vi "light_control.vi"() -> ()   [LabVIEW 2017]
uses:
  <vilib>/LabVIEW Interface for Arduino/Type Defs/Arduino Resource.ctl
  <vilib>/LabVIEW Interface for Arduino/Type Defs/Board Type.ctl
  <vilib>/LabVIEW Interface for Arduino/LabVIEW Interface for Arduino.lvlib
panel:
  in  "紫光":bool
  in  "PWM9":u8=70
  in  "PWM8":u8=70
  in  "PWM7":u8=70
  in  "PWM6":u8=70
  in  "PWM4":u8=70
  in  "PWM5":u8=70
  in  "PWM1":u8=70
  in  "PWM3":u8=70
  in  "PWM2":u8=70
  out "PWM Pins 3":u8[](array[numeric])
  out "PWM Pins 2":u8[](array[numeric])
  out "PWM Pins":u8[](array[numeric])
  out "机电控制报错1":errorcluster caption="机电控制报错"
  out "机电控制资源1":T1={"VISA resource"="", "Board Type"=enum."Uno", "Connection Type"=enum."USB / Serial", "Bytes Per Packet (15)"=15} caption="机电控制资源"
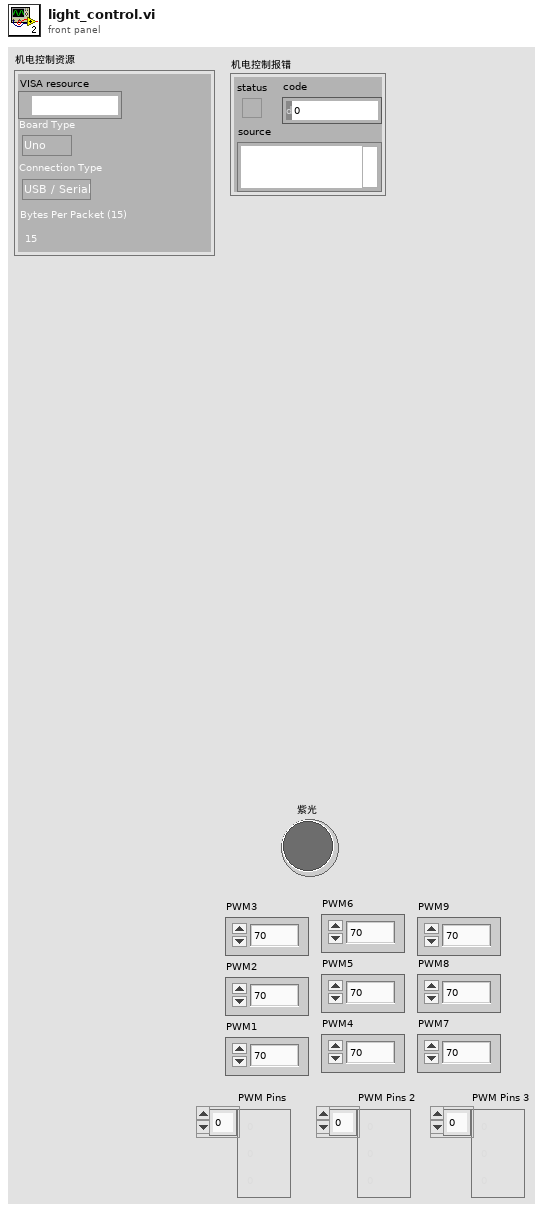
[diagram p1: front panel]
types:
  T1 = typedef "LabVIEW Interface for Arduino.lvlib/Arduino Resource.ctl" = cluster{"VISA resource":refnum<visa-resource-name>, "Board Type":T2, "Connection Type":enum8{"USB / Serial"}, "Bytes Per Packet (15)":u8}
  T2 = typedef "LabVIEW Interface for Arduino.lvlib/Board Type.ctl" = enum16{"Uno", "Dimuelanove w/Atmega 328", "Mega 2560"}
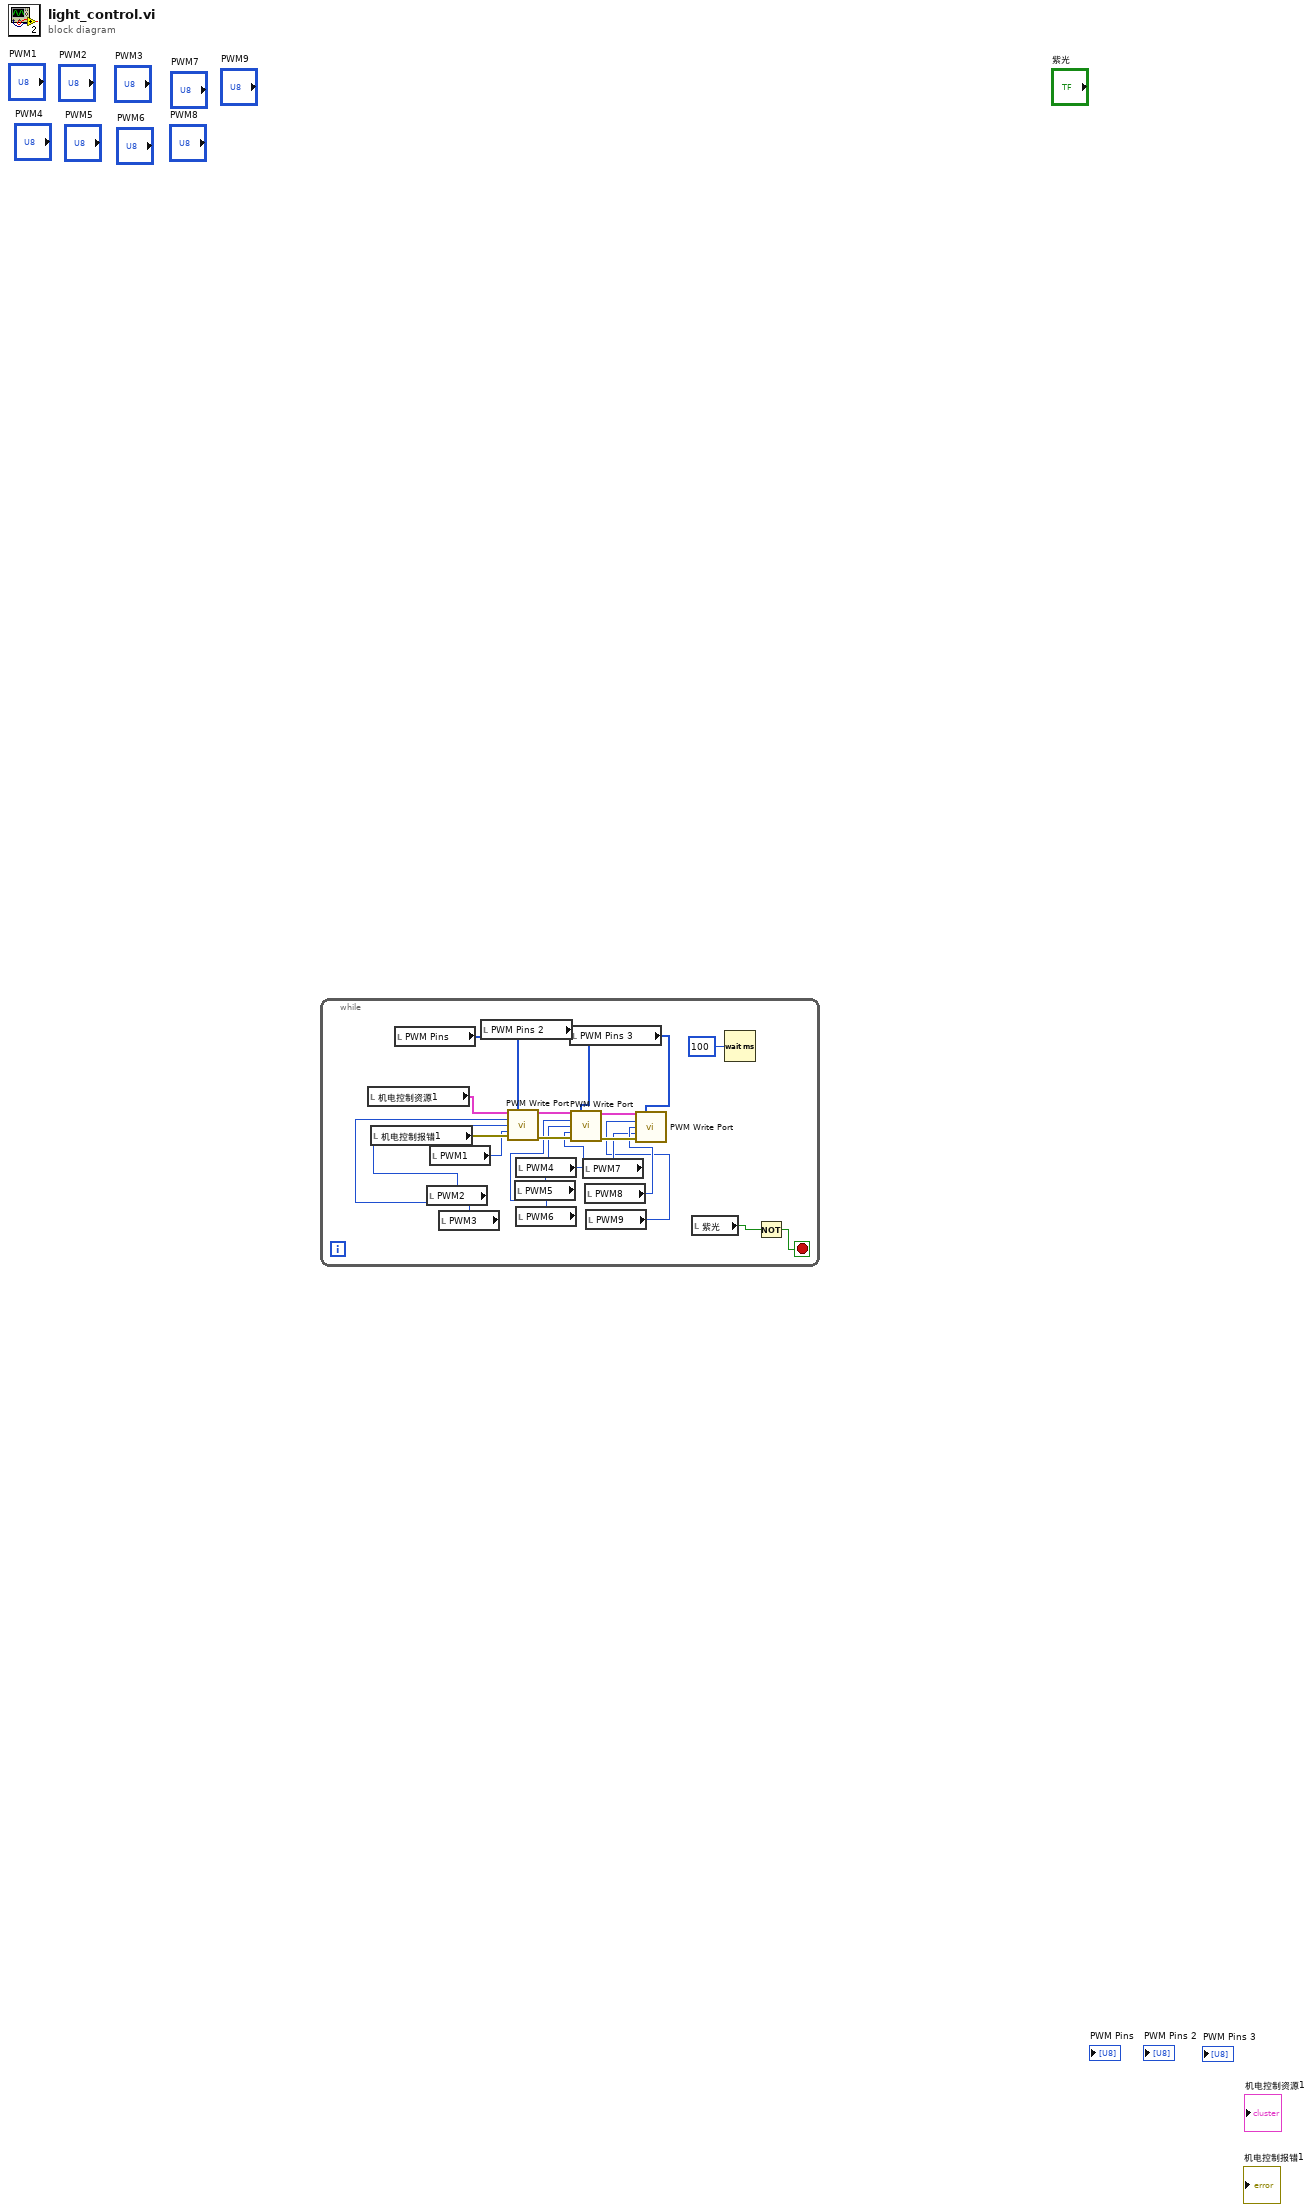
[diagram p0: block diagram]
diagram:
  n1 = while {
    stop <- w10 stop-if-true
    n2 = local read "机电控制资源1"() -> (w8:T1)
    n3 = local read "机电控制报错1"() -> (w7:errorcluster)
    n4 = local read "PWM Pins"() -> (w17:u8[])
    n5 = local read "PWM2"() -> (w12:u8)
    n6 = local read "PWM1"() -> (w6:u8)
    n7 = local read "PWM3"() -> (w5:u8)
    n8 = local read "PWM Pins 2"() -> (w16:u8[])
    n9 = call <vilib>:"PWM Write Port.vi"("Arduino Resource"=w8, "PWM Pins"=w17, "PWM 0 (0-255)"=w5, "PWM 1 (0-255)"=w12, "PWM 2 (0-255)"=w6, "error in"=w7) -> ("Arduino Resource"=w21:T1, "error out"=w20:errorcluster)  [unwired: 7 in, 1 out]
    n10 = local read "PWM5"() -> (w13:u8)
    n11 = local read "PWM4"() -> (w4:u8)
    n12 = local read "PWM6"() -> (w3:u8)
    n13 = local read "PWM Pins 3"() -> (w15:u8[])
    n14 = call <vilib>:"PWM Write Port.vi"("Arduino Resource"=w21, "PWM Pins"=w16, "PWM 0 (0-255)"=w3, "PWM 1 (0-255)"=w13, "PWM 2 (0-255)"=w4, "error in"=w20) -> ("Arduino Resource"=w19:T1, "error out"=w18:errorcluster)  [unwired: 7 in, 1 out]
    n15 = local read "PWM7"() -> (w2:u8)
    n16 = local read "PWM8"() -> (w14:u8)
    n17 = local read "PWM9"() -> (w1:u8)
    n18 = call <vilib>:"PWM Write Port.vi"("Arduino Resource"=w19, "PWM Pins"=w15, "PWM 0 (0-255)"=w1, "PWM 1 (0-255)"=w14, "PWM 2 (0-255)"=w2, "error in"=w18) -> ()  [unwired: 7 in, 3 out]
    n19 = local read "紫光"() -> (w11:bool)
    n20 = Wait (ms)(milliseconds to wait=u32 100 ("等待时间（毫秒）")) -> ()  [unwired: 1 out]
    n21 = Not(x=w11) -> (.not. x?=w10:bool)
  }
